vi "LJM_NamesToAddresses.vi"(7 "NumFrames (Auto-Detect)":i32=-1, 8 "error in":errorcluster, 11 "aNames":string[](array[string])) -> (0 "error out":errorcluster, 2 "aTypes":i32[](array[numeric]), 3 "aAddresses":i32[](array[numeric]))   [LabVIEW 2019]
panel:
  # "1/20/2015:  Default value of NumFrames changed to -1 which\nequates to Auto-Detect.  If NumFrames = -1, then the NumFrames\ncontrol is ignored and the size of aNames/aAddresses is used to\ndetermine how many frames there are."
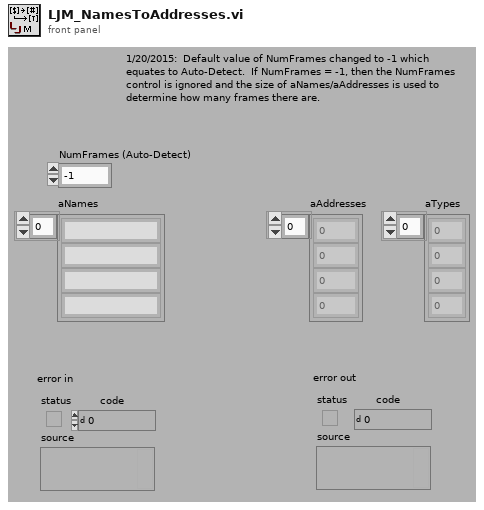
[diagram p1: front panel]
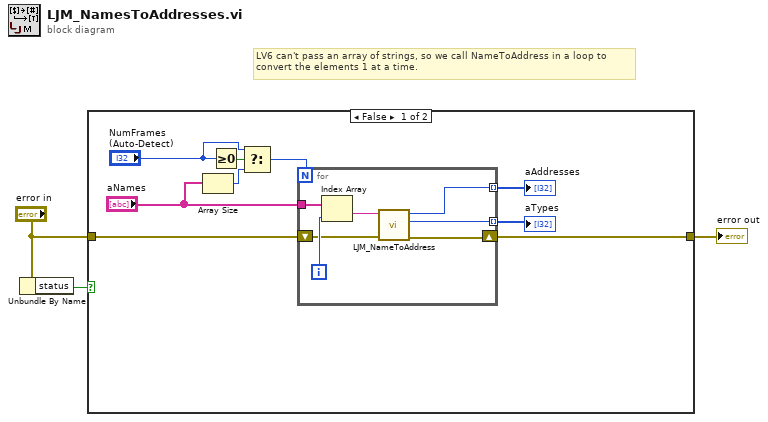
[diagram p0: block diagram]
diagram:
  # "LV6 can't pass an array of strings, so we call NameToAddress in a loop to\nconvert the elements 1 at a time."
  n1 = Unbundle By Name("error in") -> ("status"=w3:bool)
  n2 = case shown="False" w3 {
    tunnel: "error in" -> [w12 w20]
    tunnel: [w9 w20] -> w1
    frame False {
      n3 = Array Size(array="aNames") -> (size(s)=w7:i32)
      n4 = Greater Or Equal To 0?(x="NumFrames (Auto-Detect)") -> (x >= 0?=w8:bool)
      n5 = Select(t="NumFrames (Auto-Detect)", s=w8, f=w7) -> (s? t:f=w5:i32)
      n6 = for {
        N: w5 -> [_]
        tunnel: "aNames" -> [w18]
        shift-right: [w16] -> w9
        shift-left: w12 -> [w17]
        tunnel: [w14] -> w11 mode=indexing
        tunnel: [w13] -> w10 mode=indexing
        i -> [w19]
        n7 = Index Array(array=w18, index=w19) -> (element=w15:string)
        n8 = call "LJM_NameToAddress.vi"("error in"=w17, "Name"=w15) -> ("error out"=w16:errorcluster, "Type"=w14:i32, "Address"=w13:i32)  [unwired: 7 in]
      }
      "aAddresses" <- w10
      "aTypes" <- w11
    }
    frame True {
    }
  }
  "error out" <- w1
